vi "L5K Reader Action.vi"(8 "error in":errorcluster, 11 "L5K File Path":path) -> (0 "error out":errorcluster, 1 "Import Error":string, 3 "L5K Information":T1)   [LabVIEW 2011, in "Ethernet IP Custom Device Custom Device.lvlib"]
uses:
  Ethernet IP Custom Device Custom Device.lvlib
  L5K Internal Data.ctl
  L5K Tag.ctl
  L5K Data Types.ctl
  ST Enum.ctl
panel:
  in  "Import Error - String":string="\n%s - Reason: this tag is a multidimensional array. VeriStand EtherNet/IP add-on only support 1D array tags."
  in  "Import Error - Array":string="\n%s - Reason: this tag is a multidimensional array. VeriStand EtherNet/IP add-on only support 1D array tags."
  in  "Import Error - Data Type":string="\n%s - Reason: the data type of this tag is not supported by the VeriStand EtherNet/IP add-on. Enter this tag manually with a generic datatype."
  in  "Import Error":string="VeriStand EtherNet/IP add-on did not import the following tags:\n"
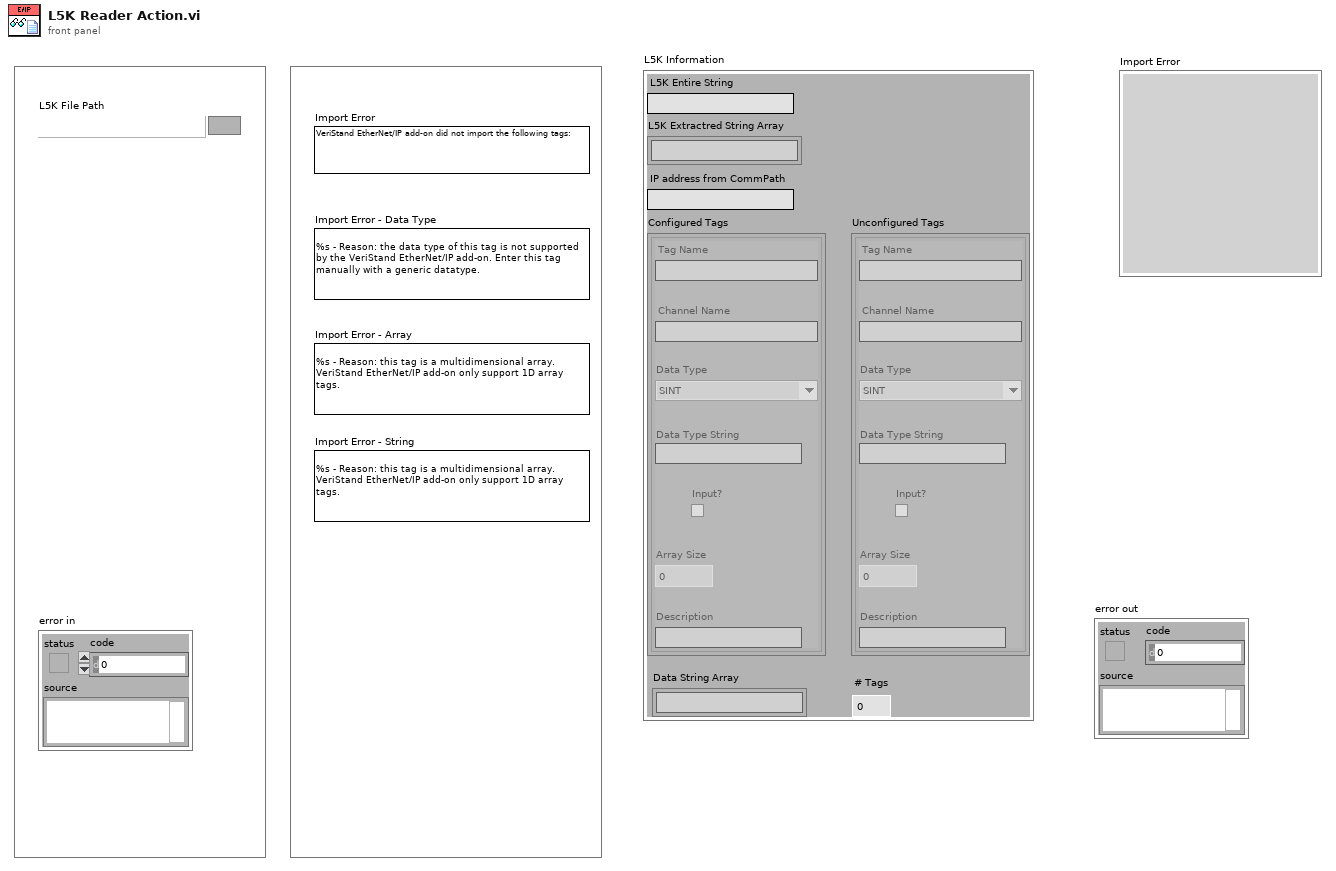
[diagram p1: front panel]
types:
  T1 = typedef "Ethernet IP Custom Device Custom Device.lvlib/L5K Internal Data.ctl" = cluster{"L5K Entire String":string, "L5K Extractred String Array":string[], "IP address from CommPath":string, "Configured Tags":T2[], "Data String Array":string[], "Unconfigured Tags":T2[], "# Tags":i32}
  T2 = typedef "Ethernet IP Custom Device Custom Device.lvlib/L5K Tag.ctl" = cluster{"Tag Name":string, "Data Type":T3, "Data Type String":string, "Array Size":i32, "Description":string, "Input?":bool, "Channel Name":string}
  T3 = typedef "Ethernet IP Custom Device Custom Device.lvlib/L5K Data Types.ctl" = enum16{"SINT", "INT", "DINT", "REAL", "BOOL"}
  T4 = typedef "Ethernet IP Custom Device Custom Device.lvlib/ST Enum.ctl" = enum16{"Init", "Extract Strings", "Extract Tags", "Exit"}
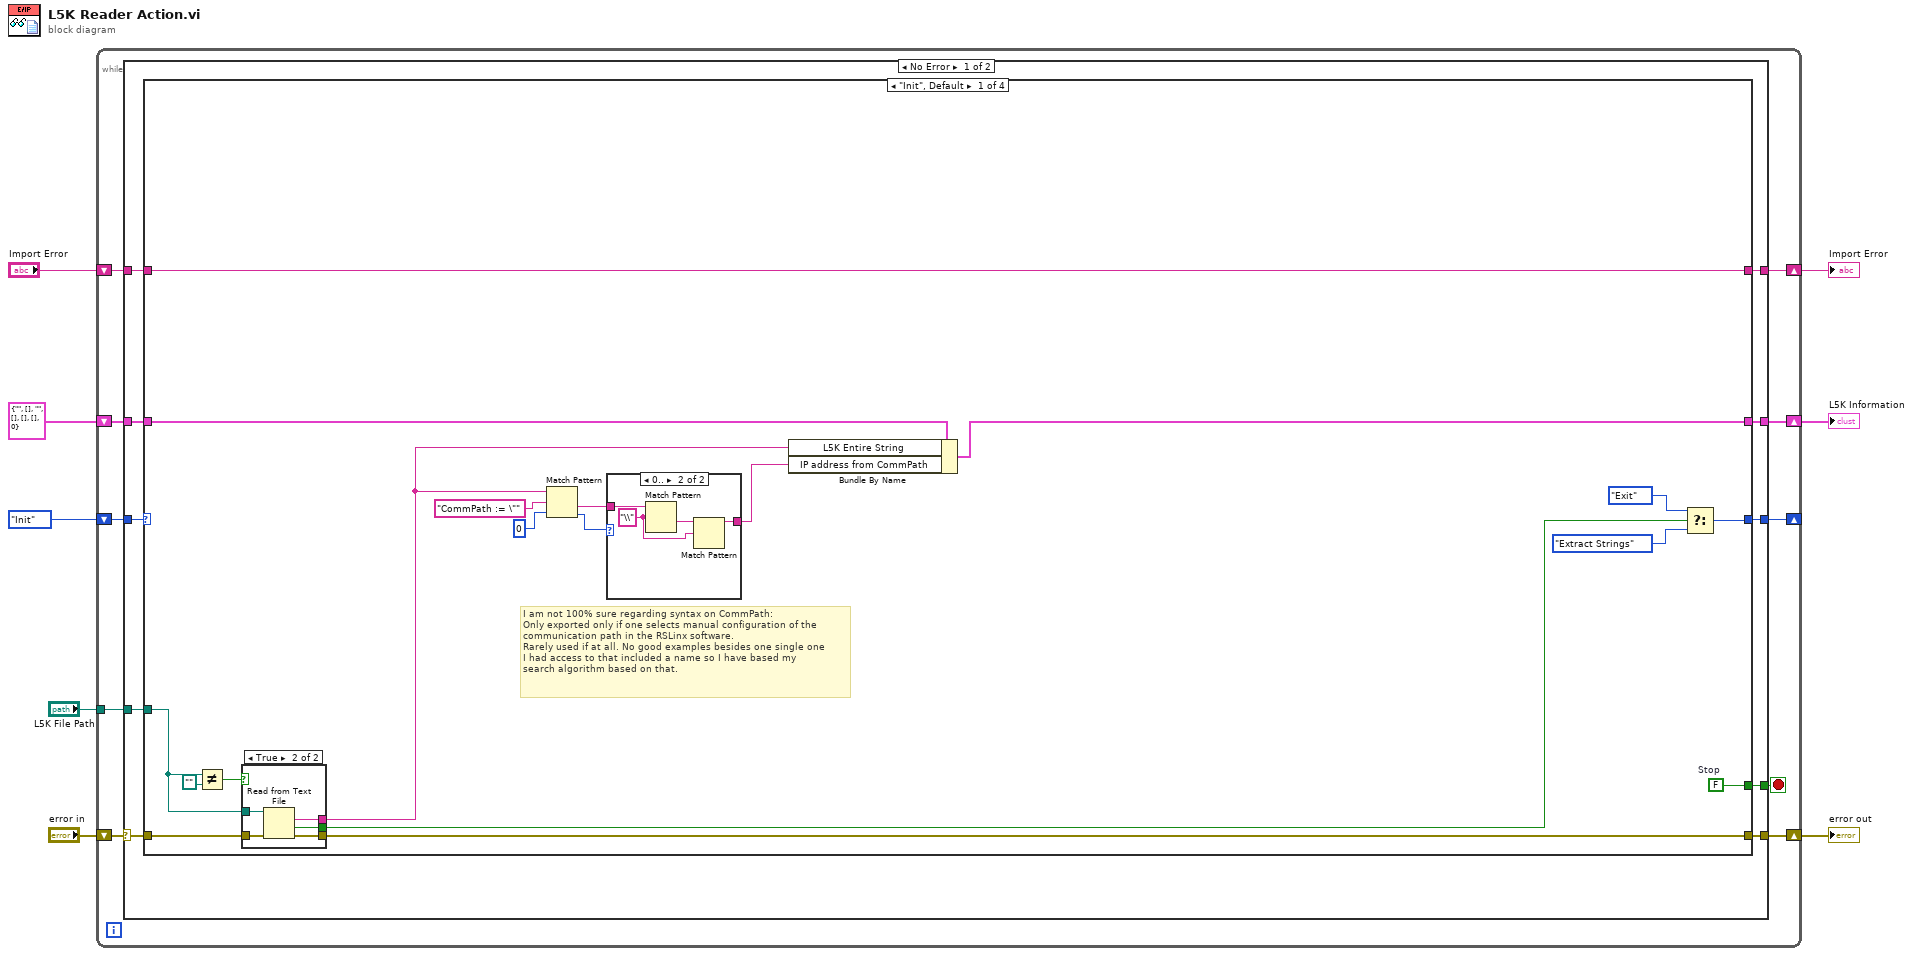
[diagram p0: block diagram]
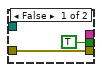
[diagram p2: hidden frame]
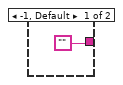
[diagram p3: hidden frame]
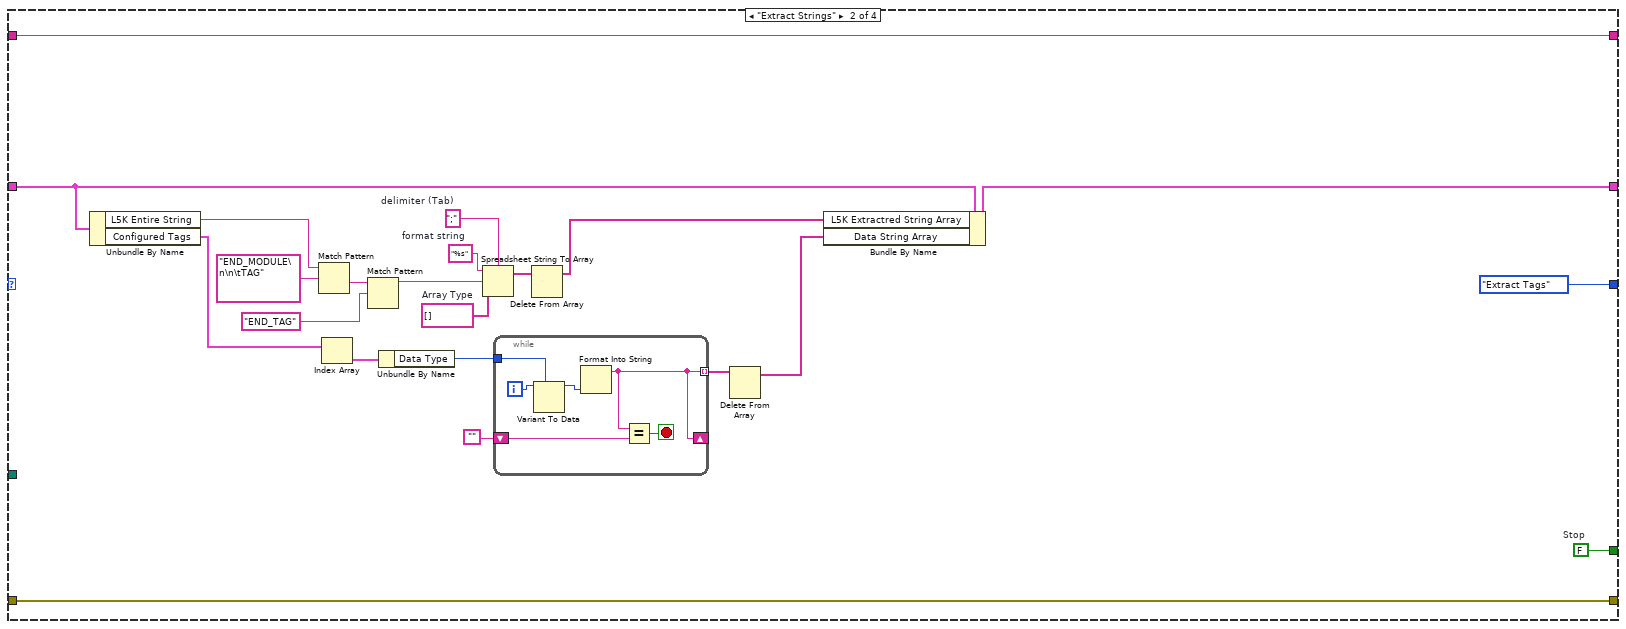
[diagram p4: hidden frame]
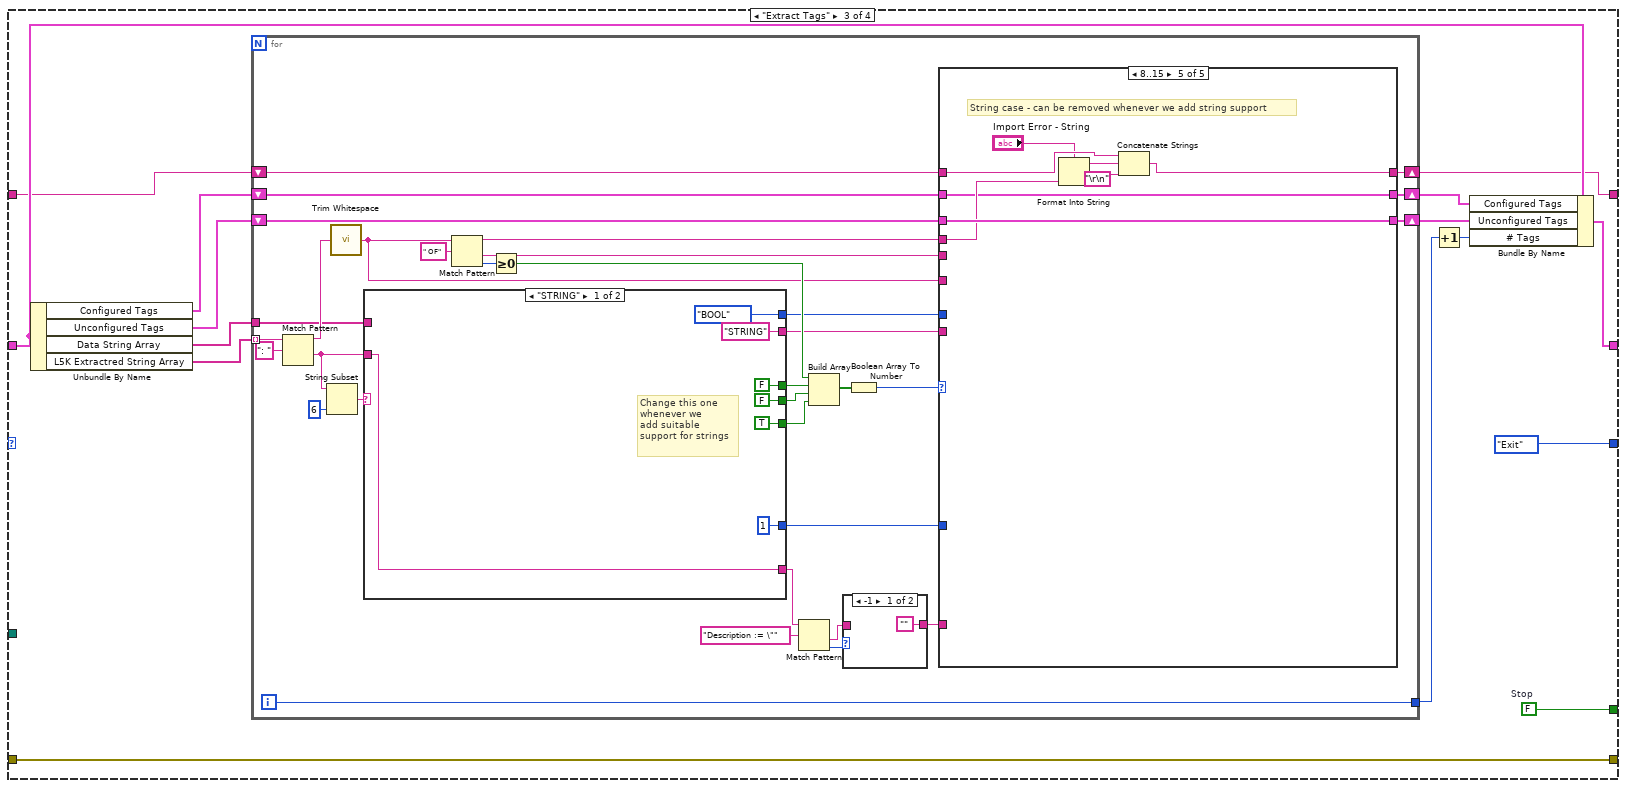
[diagram p5: hidden frame]
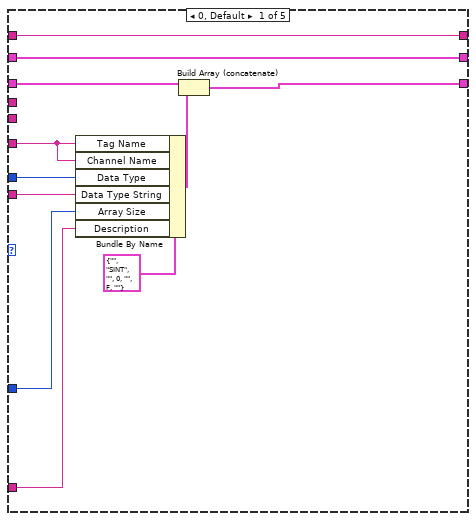
[diagram p6: hidden frame]
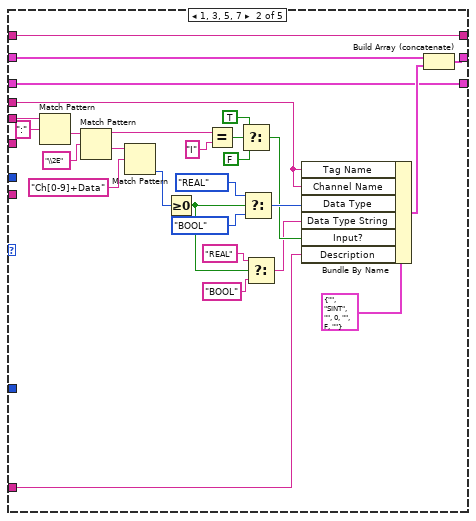
[diagram p7: hidden frame]
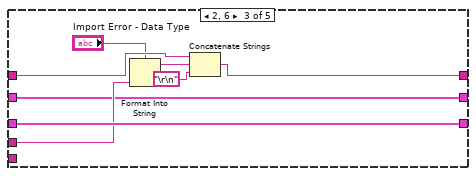
[diagram p8: hidden frame]
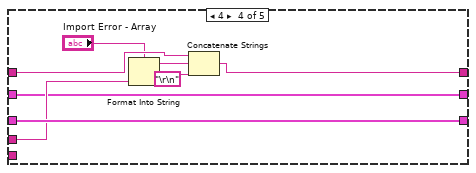
[diagram p9: hidden frame]
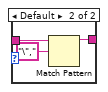
[diagram p10: hidden frame]
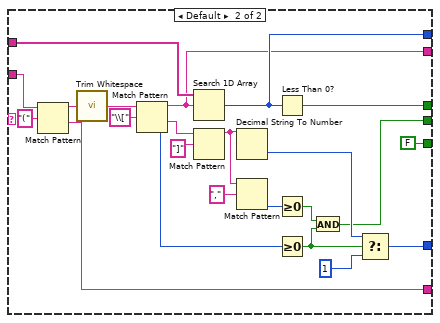
[diagram p11: hidden frame]
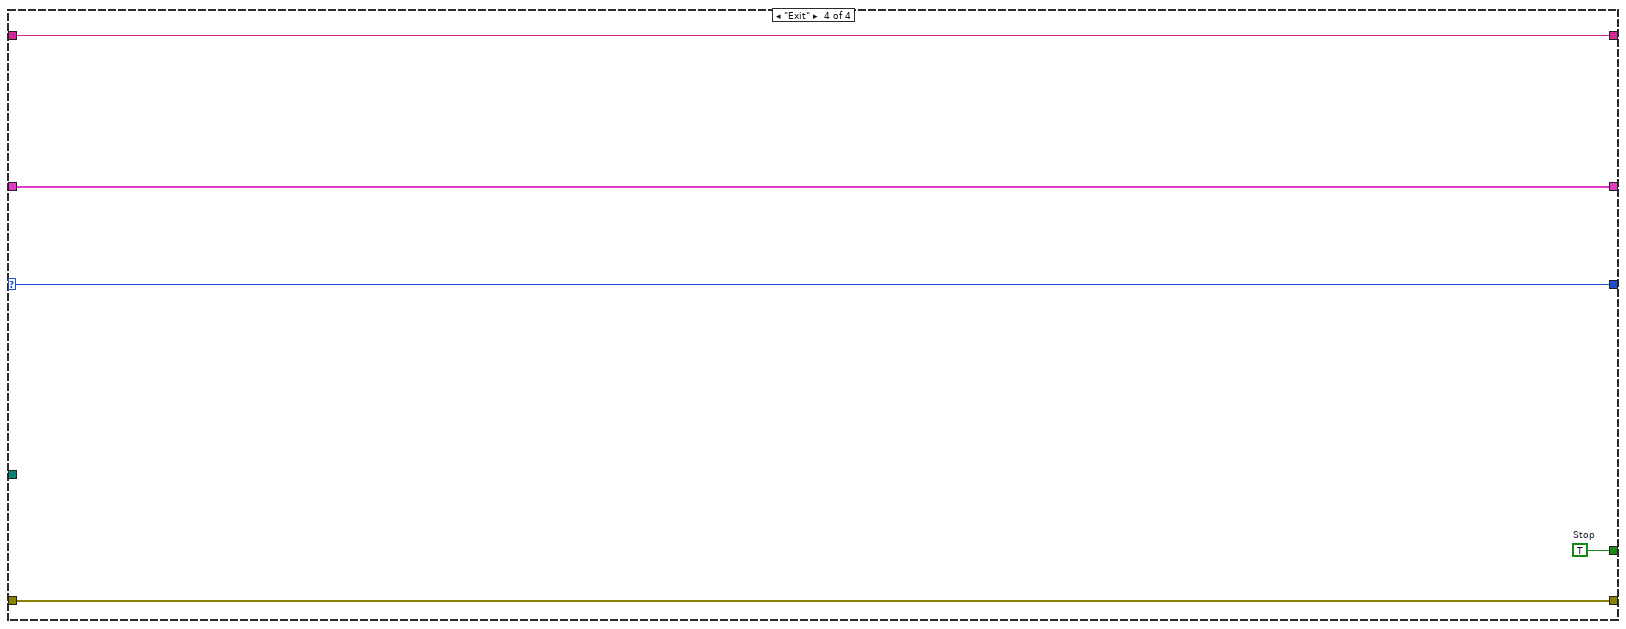
[diagram p12: hidden frame]
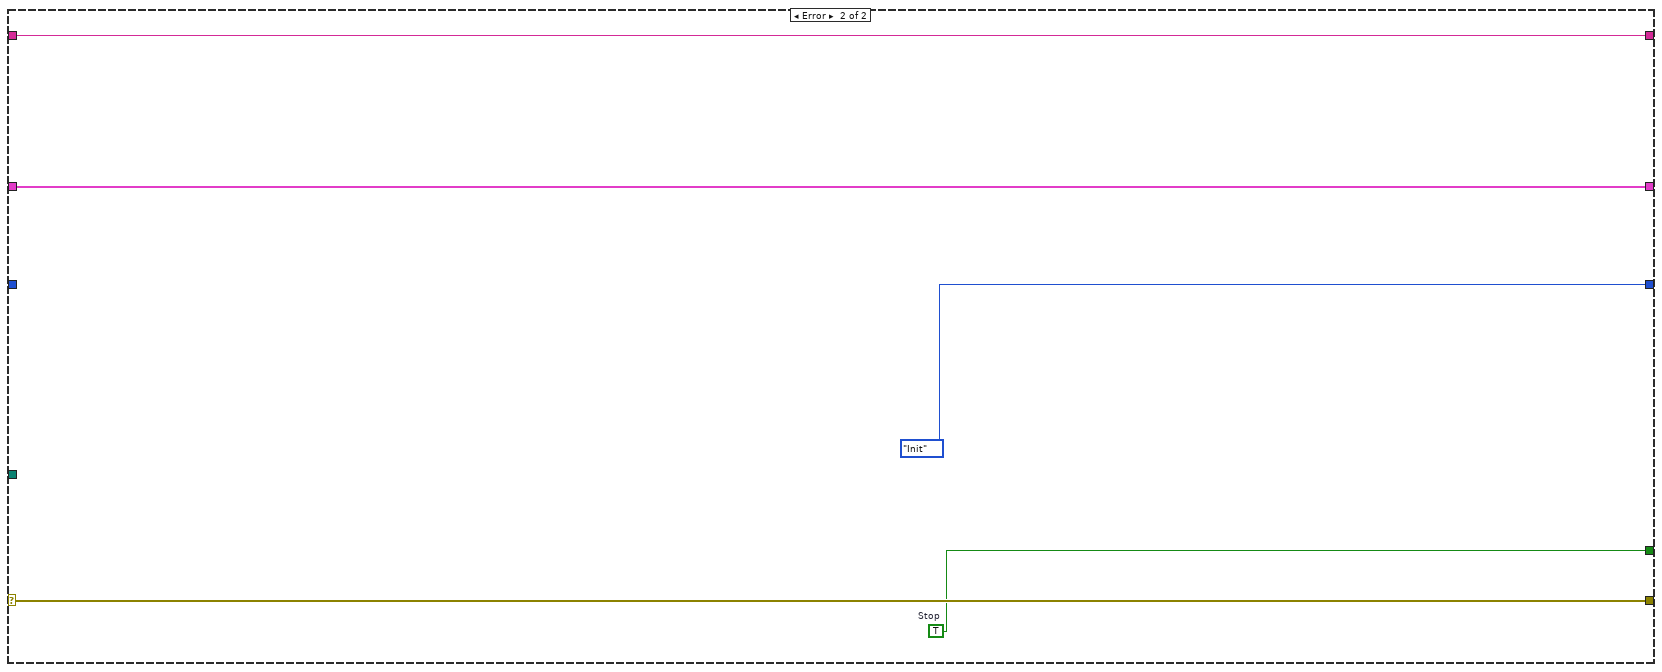
[diagram p13: hidden frame]
diagram:
  n1 = while {
    shift-right: [w16] -> _
    shift-left: ST_Enum."Init" ("Enum") -> [w18]
    shift-right: [w15] -> w5
    shift-left: "error in" -> [w12]
    shift-right: [w13] -> w1
    shift-left: T1 {"L5K Entire String"="", "L5K Extractred String Array"=[], "IP address from CommPath"="", "Configured Tags"=[], "Data String Array"=[], "Unconfigured Tags"=[], "# Tags"=0} ("L5K Information") -> [w14]
    shift-right: [w10] -> w3
    shift-left: "Import Error" -> [w11]
    tunnel: "L5K File Path" -> [w9]
    stop <- w17 stop-if-true
    n2 = case shown="No Error" w12 {
      selector: w12 -> [w22 w242]
      tunnel: w18 -> [w28 _]
      tunnel: [w27 w239] -> w17
      tunnel: [w26 ST_Enum."Init" ("Enum")] -> w16
      tunnel: [w25 w242] -> w15
      tunnel: w14 -> [w24 w241]
      tunnel: [w23 w241] -> w13
      tunnel: w11 -> [w21 w238]
      tunnel: [w20 w238] -> w10
      tunnel: w9 -> [w19 _]
      frame No Error {
        n3 = case shown="\"Init\", Default" w28 {
          selector: w28 -> [_ _ _ w236]
          tunnel: [w47 w68 w94 w237] -> w27
          tunnel: [w46 ST_Enum."Extract Tags" ("Enum") ST_Enum."Exit" ("Enum") w236] -> w26
          tunnel: w22 -> [w45 w69 w95 w235]
          tunnel: [w44 w69 w95 w235] -> w25
          tunnel: w24 -> [w43 w72 w99 w234]
          tunnel: [w42 w70 w97 w234] -> w23
          tunnel: w21 -> [w41 w60 w93 w233]
          tunnel: [w41 w60 w92 w233] -> w20
          tunnel: w19 -> [w31 _ _ _]
          frame "Init", Default {
            w47 = FALSE  # Stop
            # "I am not 100% sure regarding syntax on CommPath:\nOnly exported only if one selects manual configuration of the \ncommunication path in the RSLinx software.\nRarely used if at all. No good examples besides one single one\nI had access to that included a name so I have based my\nsearch algorithm based on that."
            n4 = Not Equal?(x=w31, y=path "") -> (x != y?=w29:bool)
            n5 = case shown="True" w29 {
              tunnel: w45 -> [w49 w54]
              tunnel: [w49 w53] -> w44
              tunnel: [TRUE ("cancelled") w52] -> w40
              tunnel: w31 -> [_ w51]
              tunnel: [_ w50] -> w33
              frame False {
              }
              frame True {
                n6 = Read from Text File(file (use dialog)=w51, error in=w54) -> (text=w50:string, cancelled=w52:bool, error out=w53:errorcluster)  [unwired: 2 in, 1 out]
              }
            }
            n7 = Match Pattern(string=w33, regular expression="CommPath := \"", offset (0)=0) -> (after substring=w36:string, offset past match=w35:i32)  [unwired: 2 out]
            n8 = case shown="0.." w35 {
              tunnel: w36 -> [_ w59]
              tunnel: ["" w56] -> w32
              frame -1, Default {
              }
              frame 0.. {
                w57 = "\\" ("regular expression")
                n9 = Match Pattern(string=w59, regular expression=w57) -> (after substring=w58:string)  [unwired: 1 in, 3 out]
                n10 = Match Pattern(string=w58, regular expression=w57) -> (before substring=w56:string)  [unwired: 1 in, 3 out]
              }
            }
            n11 = Bundle By Name(cluster=w43, "L5K Entire String"=w33, "IP address from CommPath"=w32) -> (w42:T1)
            n12 = Select(t=ST_Enum."Exit" ("Enum"), s=w40, f=ST_Enum."Extract Strings" ("Enum")) -> (s? t:f=w46:T4)
          }
          frame "Extract Strings" {
            w68 = FALSE  # Stop
            w80 = string[] []  # Array Type
            w79 = ";"  # delimiter (Tab)
            w78 = "%s"  # format string
            n13 = Unbundle By Name(w72) -> ("L5K Entire String"=w73:string, "Configured Tags"=w66:T2[])
            n14 = Match Pattern(string=w73, regular expression="END_MODULE\n\n\tTAG") -> (after substring=w75:string)  [unwired: 1 in, 3 out]
            n15 = Index Array(array=w66) -> (element=w65:T2)  [unwired: 1 in]
            n16 = Match Pattern(string=w75, regular expression="END_TAG") -> (before substring=w77:string)  [unwired: 1 in, 3 out]
            n17 = Unbundle By Name(w65) -> ("Data Type"=w63:T3)
            n18 = Spreadsheet String To Array(delimiter (Tab)=w79, format string=w78, spreadsheet string=w77, array type (2D Dbl)=w80) -> (array=w81:string[])
            n19 = while {
              shift-right: [w82] -> _
              shift-left: "" -> [w86]
              tunnel: w63 -> [w85]
              tunnel: [w82] -> w62 mode=indexing
              i -> [w84]
              stop <- w87 stop-if-true
              n20 = Variant To Data(type=w85, Variant=w84) -> (data=w83:T3)  [unwired: 1 in, 1 out]
              n21 = Format Into String(w83) -> (resulting string=w82:string)  [unwired: 3 in, 1 out]
              n22 = Equal?(x=w82, y=w86) -> (x = y?=w87:bool)
            }
            n23 = Delete From Array(array=w81) -> (array with subset deleted=w71:string[])  [unwired: 2 in, 1 out]
            n24 = Delete From Array(array=w62) -> (array with subset deleted=w61:string[])  [unwired: 2 in, 1 out]
            n25 = Bundle By Name(cluster=w72, "L5K Extractred String Array"=w71, "Data String Array"=w61) -> (w70:T1)
          }
          frame "Extract Tags" {
            w94 = FALSE  # Stop
            n26 = Unbundle By Name(w99) -> ("Configured Tags"=w91:T2[], "Unconfigured Tags"=w100:T2[], "Data String Array"=w101:string[], "L5K Extractred String Array"=w102:string[])
            n27 = for {
              tunnel: w102 -> [w132] mode=indexing
              tunnel: w101 -> [w129]
              shift-right: [w112] -> w98
              shift-left: w100 -> [w113]
              shift-right: [w110] -> w92
              shift-left: w93 -> [w109]
              shift-right: [w105] -> w90
              shift-left: w91 -> [w106]
              tunnel: [w104] -> w88
              i -> [w104]
              n28 = Match Pattern(string=w132, regular expression=": ") -> (before substring=w134:string, after substring=w130:string)  [unwired: 1 in, 2 out]
              n29 = String Subset(string=w130, length (rest)=6 ("length (rest)")) -> (substring=w131:string)  [unwired: 1 in]
              n30 = call <vilib>:"Trim Whitespace.vi"("string"=w134) -> ("trimmed string"=w117:string)  [unwired: 1 in]
              n31 = case shown="\"STRING\"" w131 {
                tunnel: w130 -> [w209 w219]
                tunnel: w129 -> [_ w217]
                tunnel: [w209 w216] -> w123
                tunnel: [FALSE w215] -> w121
                tunnel: [FALSE w214] -> w120
                tunnel: [L5K_Data_Types."BOOL" ("Data Type") w213] -> w116
                tunnel: [1 ("t") w212] -> w115
                tunnel: ["STRING" ("trimmed string") w211] -> w108
                tunnel: [TRUE FALSE] -> w103
                frame "STRING" {
                  # "Change this one\nwhenever we\nadd suitable\nsupport for strings"
                }
                frame Default {
                  n32 = Match Pattern(string=w219, regular expression="(") -> (before substring=w221:string, after substring=w216:string)  [unwired: 1 in, 2 out]
                  n33 = call <vilib>:"Trim Whitespace.vi"("string"=w221) -> ("trimmed string"=w222:string)  [unwired: 1 in]
                  n34 = Match Pattern(string=w222, regular expression="\\[") -> (before substring=w211:string, after substring=w224:string, offset past match=w228:i32)  [unwired: 1 in, 1 out]
                  n35 = Search 1D Array(1D array=w217, element=w211) -> (index of element=w213:i32)  [unwired: 1 in]
                  n36 = Match Pattern(string=w224, regular expression="]") -> (before substring=w227:string)  [unwired: 1 in, 3 out]
                  n37 = Decimal String To Number(string=w227) -> (number=w220:i32)  [unwired: 2 in, 1 out]
                  n38 = Match Pattern(string=w227, regular expression=",") -> (offset past match=w230:i32)  [unwired: 1 in, 3 out]
                  n39 = Less Than 0?(x=w213) -> (x < 0?=w214:bool)
                  n40 = Greater Or Equal To 0?(x=w230) -> (x >= 0?=w231:bool)
                  n41 = Greater Or Equal To 0?(x=w228) -> (x >= 0?=w232:bool)
                  n42 = And(x=w231, y=w232) -> (x .and. y?=w215:bool)
                  n43 = Select(t=w220, s=w232, f=1 ("t")) -> (s? t:f=w212:i32)
                }
              }
              n44 = Match Pattern(string=w117, regular expression=" OF") -> (before substring=w111:string, after substring=w107:string, offset past match=w127:i32)  [unwired: 1 in, 1 out]
              n45 = Greater Or Equal To 0?(x=w127) -> (x >= 0?=w119:bool)
              n46 = Match Pattern(string=w123, regular expression="Description := \"") -> (after substring=w124:string, offset past match=w125:i32)  [unwired: 1 in, 2 out]
              n47 = Build Array(w119, w120, w121, w103) -> (w122:bool[])
              n48 = case shown="-1" w125 {
                tunnel: ["" w201] -> w114
                tunnel: w124 -> [_ w200]
                frame -1 {
                }
                frame Default {
                  n49 = Match Pattern(string=w200, regular expression="\",") -> (before substring=w201:string)  [unwired: 1 in, 3 out]
                }
              }
              n50 = Boolean Array To Number(Boolean array=w122) -> (number=w118:u32)
              n51 = case shown="8..15" w118 {
                tunnel: w117 -> [w136 _ _ _ _]
                tunnel: w116 -> [w145 _ _ _ _]
                tunnel: w115 -> [w139 _ _ _ _]
                tunnel: w114 -> [w144 w156 _ _ _]
                tunnel: w113 -> [w143 w148 w182 w190 w198]
                tunnel: [w141 w148 w182 w190 w198] -> w112
                tunnel: w111 -> [_ w147 w178 w186 w194]
                tunnel: [w140 w174 w181 w189 w197] -> w110
                tunnel: w109 -> [w140 w174 w179 w187 w195]
                tunnel: w108 -> [w138 _ _ _ _]
                tunnel: w107 -> [_ w151 _ _ _]
                tunnel: w106 -> [w137 w150 w175 w183 w191]
                tunnel: [w137 w149 w175 w183 w191] -> w105
                frame 0, Default {
                  n52 = Bundle By Name(cluster=T2 {"Tag Name"="", "Data Type"=enum."SINT", "Data Type String"="", "Array Size"=0, "Description"="", "Input?"=FALSE, "Channel Name"=""} ("Tag"), "Tag Name"=w136, "Channel Name"=w136, "Data Type"=w145, "Data Type String"=w138, "Array Size"=w139, "Description"=w144) -> (w142:T2)
                  n53 = Build Array (concatenate)(w143, w142) -> (w141:T2[])
                }
                frame 1, 3, 5, 7 {
                  n54 = Match Pattern(string=w151, regular expression=":") -> (after substring=w169:string)  [unwired: 1 in, 3 out]
                  n55 = Match Pattern(string=w169, regular expression="\\2E") -> (before substring=w161:string, after substring=w168:string)  [unwired: 1 in, 2 out]
                  n56 = Match Pattern(string=w168, regular expression="Ch[0-9]+Data") -> (offset past match=w166:i32)  [unwired: 1 in, 3 out]
                  n57 = Greater Or Equal To 0?(x=w166) -> (x >= 0?=w155:bool)
                  n58 = Equal?(x=w161, y="I") -> (x = y?=w172:bool)
                  n59 = Select(t=TRUE, s=w172, f=FALSE) -> (s? t:f=w157:bool)
                  n60 = Select(t=L5K_Data_Types."REAL" ("Data Type"), s=w155, f=L5K_Data_Types."BOOL" ("Data Type")) -> (s? t:f=w165:T3)
                  n61 = Select(t="REAL", s=w155, f="BOOL") -> (s? t:f=w152:string)
                  n62 = Bundle By Name(cluster=T2 {"Tag Name"="", "Data Type"=enum."SINT", "Data Type String"="", "Array Size"=0, "Description"="", "Input?"=FALSE, "Channel Name"=""} ("Tag"), "Tag Name"=w147, "Channel Name"=w147, "Data Type"=w165, "Data Type String"=w152, "Input?"=w157, "Description"=w156) -> (w158:T2)
                  n63 = Build Array (concatenate)(w150, w158) -> (w149:T2[])
                }
                frame 2, 6 {
                  n64 = Format Into String(format string="Import Error - Data Type", w178) -> (resulting string=w180:string)  [unwired: 2 in, 1 out]
                  n65 = Concatenate Strings(w179, w180, "\r\n") -> (w181:string)
                }
                frame 4 {
                  n66 = Format Into String(format string="Import Error - Array", w186) -> (resulting string=w188:string)  [unwired: 2 in, 1 out]
                  n67 = Concatenate Strings(w187, w188, "\r\n") -> (w189:string)
                }
                frame 8..15 {
                  # "String case - can be removed whenever we add string support"
                  n68 = Format Into String(format string="Import Error - String", w194) -> (resulting string=w196:string)  [unwired: 2 in, 1 out]
                  n69 = Concatenate Strings(w195, w196, "\r\n") -> (w197:string)
                }
              }
            }
            n70 = Increment(x=w88) -> (x+1=w89:i32)
            n71 = Bundle By Name(cluster=w99, "Configured Tags"=w90, "Unconfigured Tags"=w98, "# Tags"=w89) -> (w97:T1)
          }
          frame "Exit" {
            w237 = TRUE  # Stop
          }
        }
      }
      frame Error {
        w239 = TRUE  # Stop
      }
    }
  }
  "error out" <- w5
  "Import Error" <- w3
  "L5K Information" <- w1
